vi "Configure Trigger Slope.vi"(8 "error in (no error)":errorcluster, 9 "Trigger Slope (0: Rising)":u16(ring) items=["Rising", "Falling"], 10 "Channel (0: Channel 1)":u16(ring) items=["Channel 1", "Channel 2", "Channel 3", "Channel 4", "EX", "EX10", "Line"], 11 "VISA resource name":refnum<visa-resource-name>) -> (0 "error out":errorcluster, 3 "VISA resource name out":refnum<visa-resource-name>)   [LabVIEW 2015, in "LeCroy Wave Series.lvlib"]
doc: "Sets the trigger slope of the specified trigger source."
uses:
  <instrlib>/LeCroy Wave Series/LeCroy Wave Series.lvlib
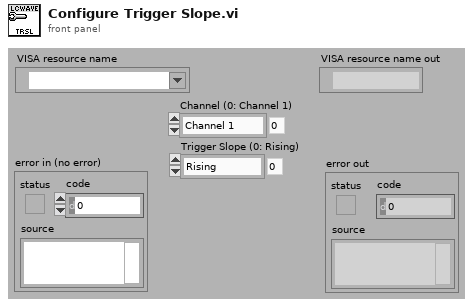
[diagram p1: front panel]
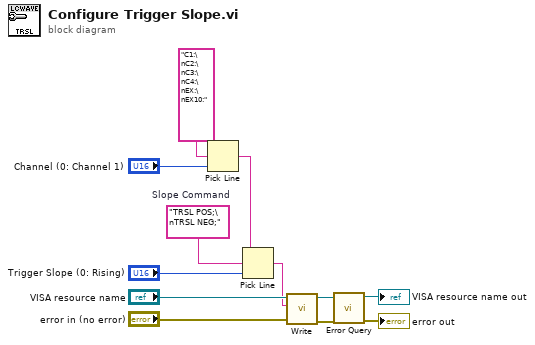
[diagram p0: block diagram]
diagram:
  w12 = "TRSL POS;\nTRSL NEG;"  # Slope Command
  n1 = Pick Line(multi-line string="C1:\nC2:\nC3:\nC4:\nEX:\nEX10:", line index="Channel (0: Channel 1)") -> (output string=w6:string)  [unwired: 1 in]
  n2 = Pick Line(string ("")=w6, multi-line string=w12, line index="Trigger Slope (0: Rising)") -> (output string=w5:string)
  n3 = call <instrlib>:"Write.vi"("error in (no error)"="error in (no error)", "Write Buffer"=w5, "VISA resource name"="VISA resource name") -> ("error out"=w1:errorcluster, "VISA resource name out"=w4:refnum<visa-resource-name>)  [unwired: 6 in, 1 out]
  n4 = call <instrlib>:"Error Query.vi"("error in (no error)"=w1, "VISA resource name"=w4) -> ("error out"=→"error out":errorcluster, "VISA resource name out"=→"VISA resource name out":refnum<visa-resource-name>)  [unwired: 6 in, 2 out]
